vi "Create Dvr.vi"(8 "Error In":errorcluster, 11 "NumericOperation in":refnum<class "NumericOperation.lvclass">) -> (0 "Error Out":errorcluster, 2 "Data Value Reference":refnum<data-value>, 3 "NumericOperation out":refnum<class "NumericOperation.lvclass">)   [LabVIEW 2021, in "Calculator.lvlib" / "NumericOperation.lvclass"]
doc: "This VI creates a Data Value Reference of the input datatype."
uses:
  NumericOperation.lvclass
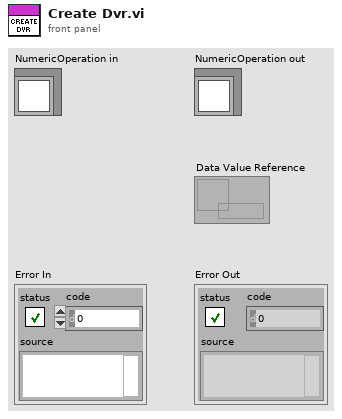
[diagram p1: front panel]
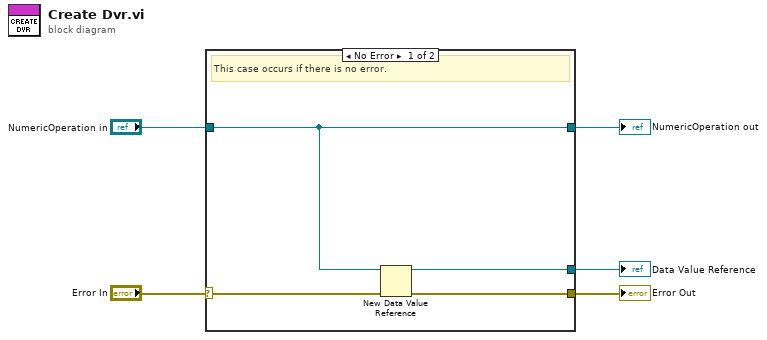
[diagram p0: block diagram]
diagram:
  n1 = case shown="No Error" "Error In" {
    selector: "Error In" -> [w7 w11]
    tunnel: [w6 w11] -> w4
    tunnel: [w9 w10] -> w2
    tunnel: "NumericOperation in" -> [w9 w10]
    tunnel: [w8 _] -> w1
    frame No Error {
      # "This case occurs if there is no error."
      n2 = New Data Value Reference(data value=w9, error in=w7) -> (data value reference=w8:refnum<data-value>, error out=w6:errorcluster)
    }
    frame Error {
      # "This case occurs if there is any error."
    }
  }
  "Error Out" <- w4
  "NumericOperation out" <- w2
  "Data Value Reference" <- w1
